vi "Select_Alternative_channel.vi"(4 "Filetype":string, 5 "All Tabulated Channels":string[](array[string]), 6 "Reading Filename":path, 7 "Start of data (bytes)":i32, 8 "Template Channel Name":string, 9 "Data string":string, 10 "Previous Channels used":string[](array[string])) -> (0 "Choosen Channel":string, 3 "Selected Index":i32)   [LabVIEW 2010]
uses:
  Results_plotter_Global.vi
panel:
  out "Channel Values":dbl[](graph)
  out "Channel Values":string[](array[string])
  out "Message":string
  in  "Boolean":bool
  in  "Select channel to be used":u16(ring) items=["No Suitable Channel Found", "No Suitable Channel Found, Don't Prompt again", "::X [mm]", "::Y [mm]", "::Z [mm]", "::Uo", "::Ur", "::U", "::u^2", "::Ur/Uo", "::U/Ur", "::u^2/Ur^2", "::z/delta", "Measurement:Type:", "::Comments", "BL:Depth:[mm]", "Date:of:Measurement", "Current:Data:Filename", "Current:Data File:1st Folder level", "Current:Data File:2nd Folder level", "Current:Data File:3rd Folder level", "Current:Data File:4th Folder level", "Current:File:Number"]
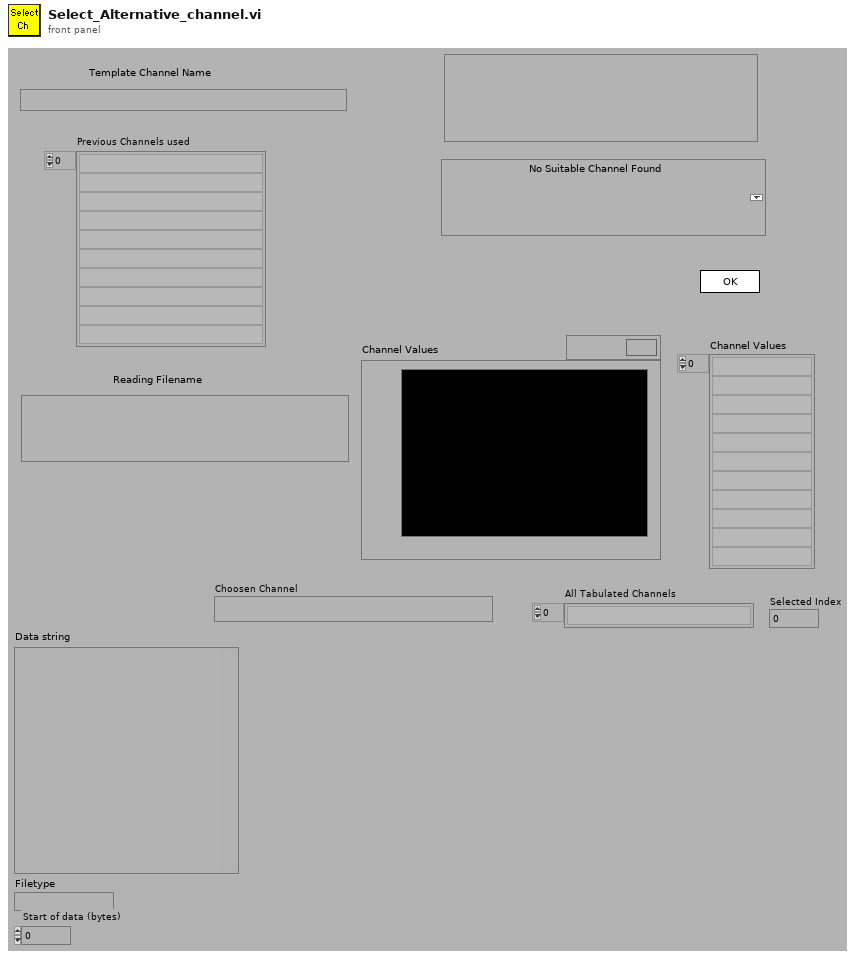
[diagram p1: front panel]
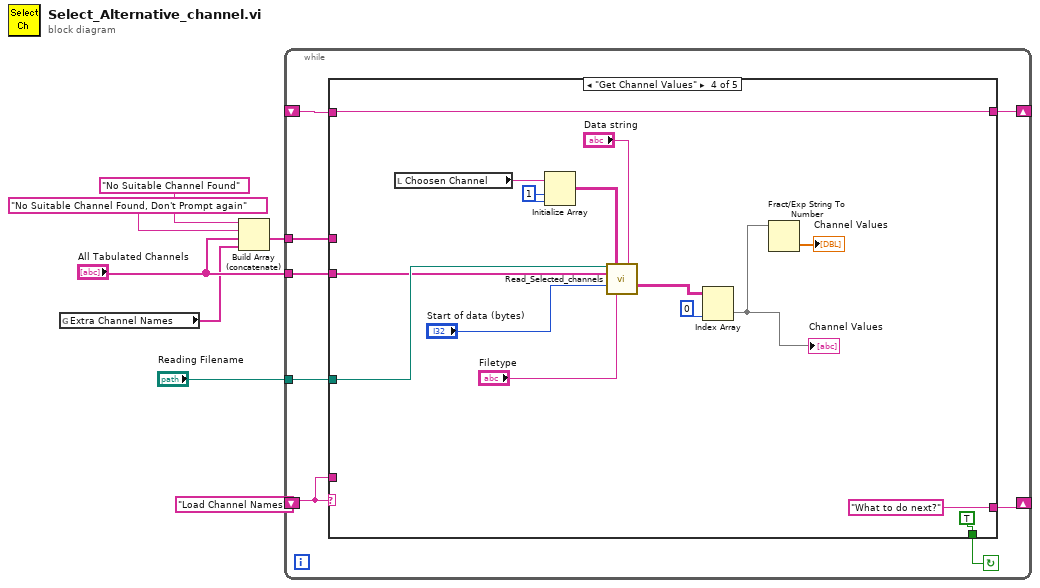
[diagram p0: block diagram]
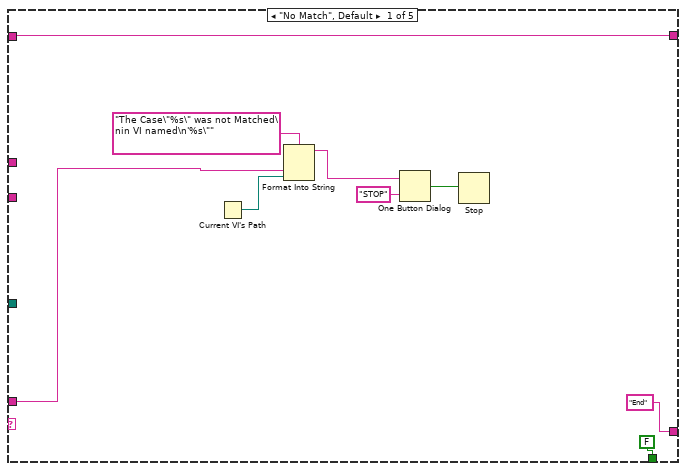
[diagram p2: hidden frame]
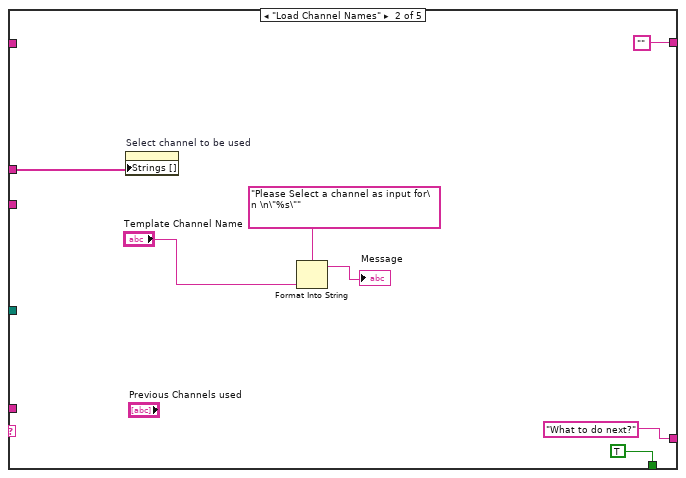
[diagram p3: hidden frame]
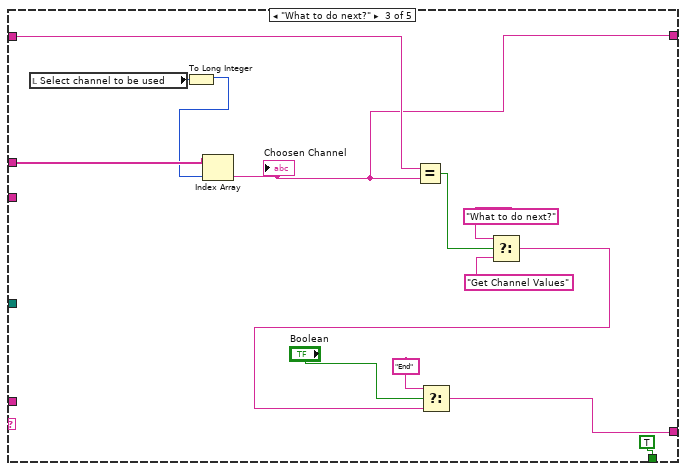
[diagram p4: hidden frame]
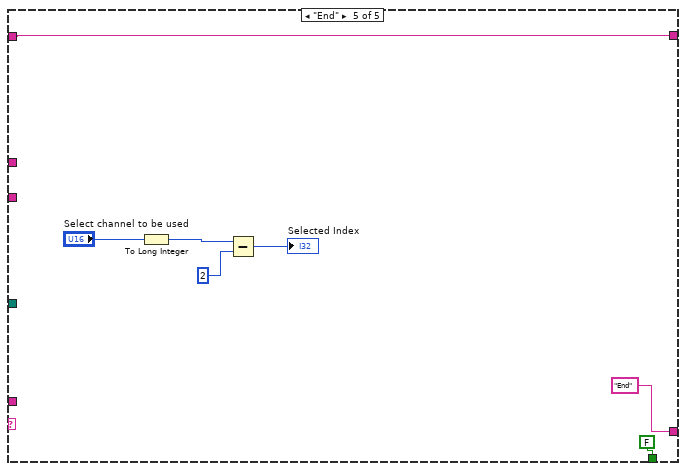
[diagram p5: hidden frame]
diagram:
  n1 = global read "Results_plotter_Global.vi" "Extra Channel Names"() -> (w1:string[])
  n2 = Build Array (concatenate)("No Suitable Channel Found" ("Input Element"), "No Suitable Channel Found, Don't Prompt again" ("Input Element"), "All Tabulated Channels", w1) -> (w5:string[])
  n3 = while {
    tunnel: w5 -> [w14]
    shift-left: "Load Channel Names" -> [w12]
    shift-right: [w13] -> _
    tunnel: "Reading Filename" -> [w11]
    tunnel: "All Tabulated Channels" -> [w10]
    shift-right: [w8] -> _
    shift-left: _ -> [w9]
    stop <- w15 continue-if-true
    n4 = case shown="\"Get Channel Values\"" w12 {
      tunnel: [FALSE TRUE TRUE TRUE FALSE] -> w15
      tunnel: w14 -> [_ w30 w39 _ _]
      tunnel: ["End" "What to do next?" w41 "What to do next?" "End"] -> w13
      tunnel: w12 -> [w19 _ _ _ _]
      tunnel: w11 -> [_ _ _ w58 _]
      tunnel: w10 -> [_ _ _ w57 _]
      tunnel: w9 -> [w16 _ w37 w46 w61]
      tunnel: [w16 "" w36 w46 w61] -> w8
      frame "No Match", Default {
        n5 = Current VI's Path() -> (path=w24:path)
        n6 = Format Into String(format string="The Case\"%s\" was not Matched\nin VI named\n'%s\"" ("Format String"), w19, w24) -> (resulting string=w21:string)  [unwired: 2 in, 1 out]
        n7 = One Button Dialog(message=w21, button name ("OK")="STOP") -> (true=w23:bool)
        n8 = Stop(stop? (T)=w23) -> ()
      }
      frame "Load Channel Names" {
        n9 = property on="Select channel to be used" class="Ring (strict)"("Strings []"=w30) -> ()  [unwired: 2 in, 2 out]
        n10 = Format Into String(format string="Please Select a channel as input for\n \n\"%s\"" ("Format String"), "Template Channel Name") -> (resulting string=→"Message":string)  [unwired: 2 in, 1 out]
      }
      frame "What to do next?" {
        n11 = local read "Select channel to be used"() -> (w44:u16)
        n12 = To Long Integer(number=w44) -> (32bit integer=w38:i32)
        n13 = Index Array(array=w39, index=w38) -> (element=w36:string)
        "Choosen Channel" <- w36
        n14 = Equal?(x=w37, y=w36) -> (x = y?=w33:bool)
        n15 = Select(t="What to do next?", s=w33, f="Get Channel Values") -> (s? t:f=w32:string)
        n16 = Select(t="End", s="Boolean", f=w32) -> (s? t:f=w41:string)
      }
      frame "Get Channel Values" {
        w55 = 1 ("dimension size")
        n17 = local read "Choosen Channel"() -> (w56:string)
        n18 = Initialize Array(w56, w55, w55) -> (w54:string[][])
        n19 = call "Read_Selected_channels.vi"("Filename"=w58, "Valid Channel Options"=w54, "Data string"="Data string", "All Channels Present"=w57, "Start of data (bytes)"="Start of data (bytes)", "Filetype"="Filetype") -> ("Output Values"=w50:string[][])  [unwired: 4 in, 5 out]
        n20 = Index Array(array=w50, index (col)=0 ("index (row)")) -> (element=w49:string[])  [unwired: 1 in]
        "Channel Values" <- w49
        n21 = Fract/Exp String To Number(string=w49) -> (number=→"Channel Values":dbl[])  [unwired: 4 out]
      }
      frame "End" {
        n22 = To Long Integer(number="Select channel to be used") -> (32bit integer=w60:i32)
        n23 = Subtract(x=w60, y=2) -> (x-y=→"Selected Index":i32)
      }
    }
  }
